vi "FGV_Preis.vi"(7 "fgv-Status":T1, 8 "error in (no error)":errorcluster, 10 "Preis Input":dbl format="%#_13g") -> (0 "error out":errorcluster, 2 "Preis Output":dbl)   [LabVIEW 2023]
doc: "FGV Preis"
uses:
  CONTROLS/FGV-status.ctl
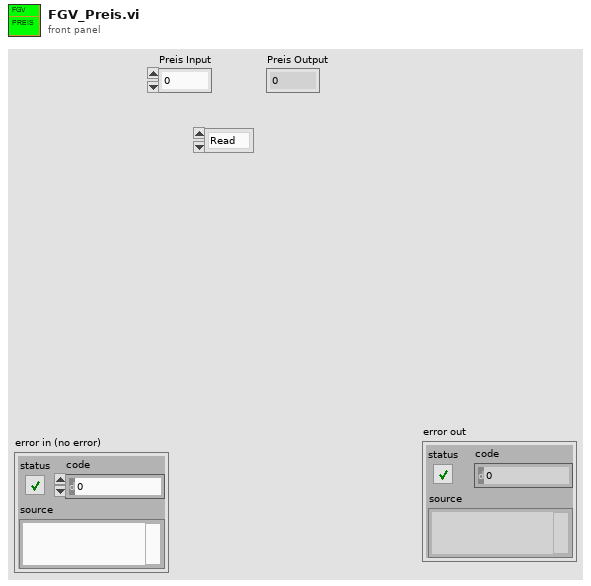
[diagram p1: front panel]
types:
  T1 = typedef "FGV-status.ctl" = enum16{"Read", "Write"}
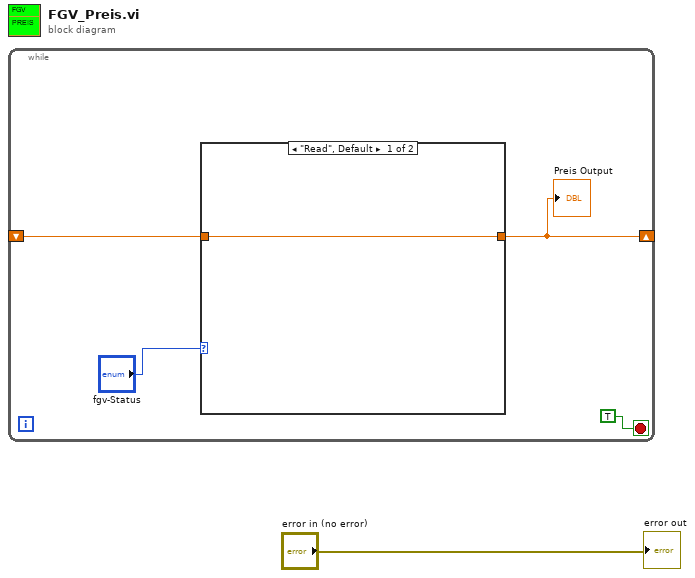
[diagram p0: block diagram]
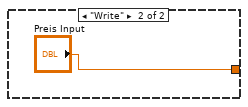
[diagram p2: hidden frame]
diagram:
  n1 = while {
    shift-right: [w2] -> _
    shift-left: _ -> [w3]
    stop <- TRUE stop-if-true
    n2 = case shown="\"Read\", Default" "fgv-Status" {
      tunnel: [w6 "Preis Input"] -> w2
      tunnel: w3 -> [w6 _]
      frame "Read", Default {
      }
      frame "Write" {
      }
    }
    "Preis Output" <- w2
  }
  "error out" <- "error in (no error)"
